vi "Read Data.vi"(6 "chip select (1st chip)":enum16{"1st chip", "2nd chip"}(ring), 8 "error in (no error)":errorcluster, 11 "LCD in":u32) -> (0 "error out":errorcluster, 1 "data":u8=97 format="%.0x", 3 "LCD out":u32)   [LabVIEW 2015, in "HD44780 FPGA.lvlib"]
doc: "Reads data at the current address from character LCD devices. The address moves according to the entry mode after you call this VI. This VI does not shift the display."
uses:
  <vilib>/EmbeddedDisplay/Hitachi HD44780/FPGA/HD44780 FPGA.lvlib
  <vilib>/EmbeddedDisplay/Hitachi HD44780/Common/HD44780 Common.lvlib
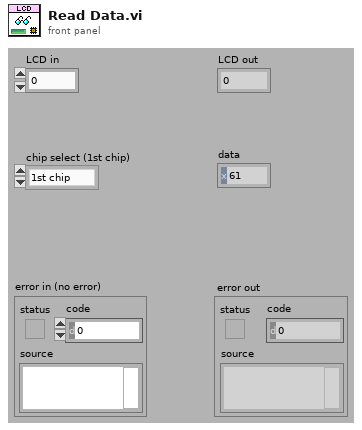
[diagram p1: front panel]
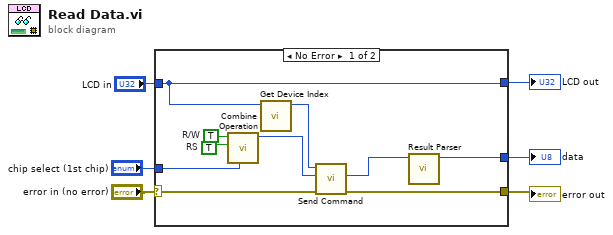
[diagram p0: block diagram]
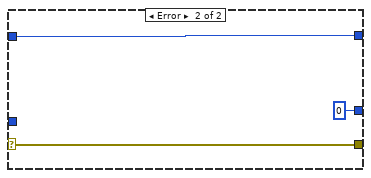
[diagram p2: hidden frame]
diagram:
  n1 = case shown="No Error" "error in (no error)" {
    selector: "error in (no error)" -> [w13 w19]
    tunnel: [w12 w19] -> w5
    tunnel: "LCD in" -> [w7 w18]
    tunnel: "chip select (1st chip)" -> [w11 _]
    tunnel: [w7 w18] -> w2
    tunnel: [w9 u8 0 ("data")] -> w1
    frame No Error {
      w15 = TRUE  # R/W
      w16 = TRUE  # RS
      n2 = call <vilib>:"Combine Operation.vi"("chip select  (1st chip)"=w11, "RS"=w16, "R/W"=w15) -> ("output"=w14:u32)  [unwired: 8 in]
      n3 = call <vilib>:"Get Device Index.vi"("LCD in"=w7) -> ("device index"=w8:i8)  [unwired: 10 in]
      n4 = call <vilib>:"Send Command.vi"("error in (no error)"=w13, "operation"=w14, "device index"=w8) -> ("error out"=w12:errorcluster, "Result"=w10:u32)  [unwired: 6 in, 1 out]
      n5 = call <vilib>:"Result Parser.vi"("operation"=w10) -> ("data"=w9:u8)  [unwired: 8 in, 2 out]
    }
    frame Error {
    }
  }
  "error out" <- w5
  "LCD out" <- w2
  "data" <- w1
